vi "arreglo4.vi"() -> ()   [LabVIEW 2011]
panel:
  in  "SALIR":bool
  in  "BSUMA":bool
  out "MENOR":dbl
  out "MAYOR":dbl
  out "PROMEDIO":dbl
  out "SUMA":dbl
  out "Array":dbl[](array[numeric])
  in  "GENERAR":bool
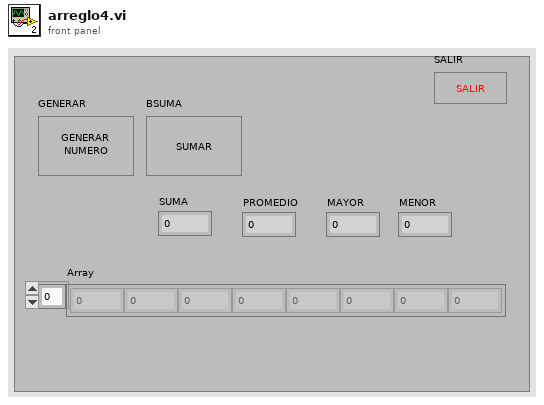
[diagram p1: front panel]
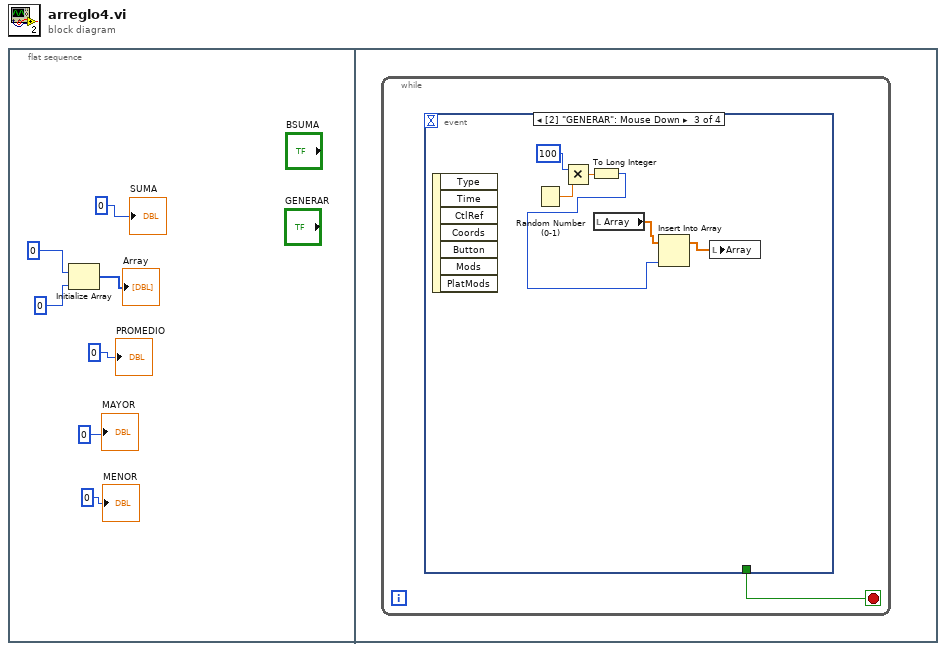
[diagram p0: block diagram]
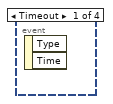
[diagram p2: hidden frame]
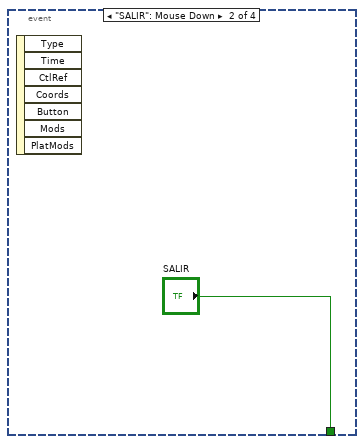
[diagram p3: hidden frame]
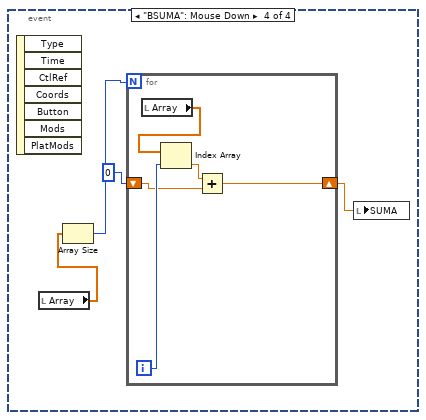
[diagram p4: hidden frame]
diagram:
  n1 = flat-sequence {
    frame #0 {
      n2 = Initialize Array(0, 0) -> (→"Array":i32[])
      "SUMA" <- 0
      "PROMEDIO" <- 0
      "MAYOR" <- 0
      "MENOR" <- 0
    }
    frame #1 {
      n3 = while {
        stop <- w8 stop-if-true
        n4 = event shown="[2] \"GENERAR\": Mouse Down" {
          selector: _ -> [_ _ _ _]
          dyn-events: _ -> [_ _ _ _]
          timeout: _ -> [_ _ _ _]
          tunnel: [_ "SALIR" _ _] -> w8
          event Timeout {
            n5 = event-data() -> ()  [unwired: 1 in, 2 out]
          }
          event "SALIR": Mouse Down {
            n6 = event-data() -> ()  [unwired: 1 in, 7 out]
          }
          event "GENERAR": Mouse Down {
            n7 = event-data() -> ()  [unwired: 1 in, 7 out]
            n8 = Random Number (0-1)() -> (number: 0 to 1=w15:dbl)
            n9 = Multiply(x=100, y=w15) -> (x*y=w13:dbl)
            n10 = To Long Integer(number=w13) -> (32bit integer=w11:i32)
            n11 = local read "Array"() -> (w12:dbl[])
            n12 = Insert Into Array "Insert Into Array"(array=w12, new element=w11) -> (w10:dbl[])  [unwired: 1 in]
            n13 = local write "Array"(w10) -> ()
          }
          event "BSUMA": Mouse Down {
            n14 = event-data() -> ()  [unwired: 1 in, 7 out]
            n15 = local read "Array"() -> (w16:dbl[])
            n16 = Array Size(array=w16) -> (size(s)=w19:i32)
            n17 = for {
              N: w19 -> [_]
              shift-right: [w20] -> w17
              shift-left: 0 -> [w21]
              i -> [w24]
              n18 = local read "Array"() -> (w23:dbl[])
              n19 = Index Array(array=w23, index=w24) -> (element=w22:dbl)
              n20 = Add(x=w22, y=w21) -> (x+y=w20:dbl)
            }
            n21 = local write "SUMA"(w17) -> ()
          }
        }
      }
    }
  }
